vi "ER2007 Take Data Popup Panel.vi"() -> ()   [LabVIEW 2013]
uses:
  Controls/Global ER2007.vi
panel:
  in  "Comment":string
  in  "Delta P :":dbl format="%.2f"
  in  "Mark Options":T1(radio)
  in  "OK":bool
  in  "Pore Volume :":dbl format="%.4f"
  out "Amplitude :":dbl format="%.1f"
  out "Frequency :":dbl format="%#_0f"
  in  "Cancel":bool
  out "Cell Number :":string="<none>"
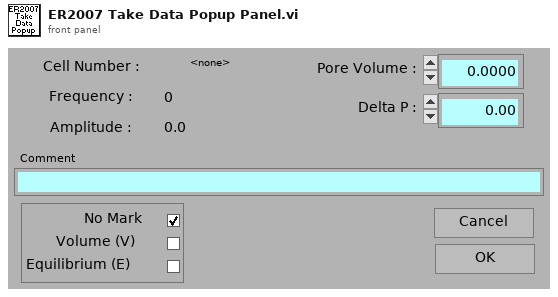
[diagram p1: front panel]
types:
  T1 = enum32{"No Mark", "Volume (V)", "Equilibrium (E)"}
  T2 = cluster{"CurCell":i32, "Cell Data":cluster{"Cell ID":i32, "Cell Status":enum16{"Inactive", "Setup", "Active", "Done"}, "Project":string, "Sample #":string, "Rock Type":string, "Fluid Pair":string, "Rw":dbl, "Rw Temp":dbl, "Length":dbl, "Diameter":dbl, "Porosity":dbl, "Permeability":dbl, "4P":bool, "ElectSpace":dbl, "Frequency":dbl, "Amplitude":dbl, "DAQ Period":u32, "DAQ Units":u16, "Start Time":dbl, "Next Time":dbl, "Datafile":path, "Last Pore Vol":dbl, "Last Pore Xdcr":enum16{"<none>", "Lo Range", "Hi Range"}, "Last Resistor":enum16{"<none>", "Resistor 1", "Resistor 2", "Resistor 3", "Resistor 4", "Resistor 5", "Resistor 6"}, "CurData":dbl[][], "Comment":string}[]}
  T3 = cluster{"Cell ID":i32, "Cell Status":enum16{"Inactive", "Setup", "Active", "Done"}, "Project":string, "Sample #":string, "Rock Type":string, "Fluid Pair":string, "Rw":dbl, "Rw Temp":dbl, "Length":dbl, "Diameter":dbl, "Porosity":dbl, "Permeability":dbl, "4P":bool, "ElectSpace":dbl, "Frequency":dbl, "Amplitude":dbl, "DAQ Period":u32, "DAQ Units":u16, "Start Time":dbl, "Next Time":dbl, "Datafile":path, "Last Pore Vol":dbl, "Last Pore Xdcr":enum16{"<none>", "Lo Range", "Hi Range"}, "Last Resistor":enum16{"<none>", "Resistor 1", "Resistor 2", "Resistor 3", "Resistor 4", "Resistor 5", "Resistor 6"}, "CurData":dbl[][], "Comment":string}[]
  T4 = cluster{"Cell ID":i32, "Cell Status":enum16{"Inactive", "Setup", "Active", "Done"}, "Project":string, "Sample #":string, "Rock Type":string, "Fluid Pair":string, "Rw":dbl, "Rw Temp":dbl, "Length":dbl, "Diameter":dbl, "Porosity":dbl, "Permeability":dbl, "4P":bool, "ElectSpace":dbl, "Frequency":dbl, "Amplitude":dbl, "DAQ Period":u32, "DAQ Units":u16, "Start Time":dbl, "Next Time":dbl, "Datafile":path, "Last Pore Vol":dbl, "Last Pore Xdcr":enum16{"<none>", "Lo Range", "Hi Range"}, "Last Resistor":enum16{"<none>", "Resistor 1", "Resistor 2", "Resistor 3", "Resistor 4", "Resistor 5", "Resistor 6"}, "CurData":dbl[][], "Comment":string}
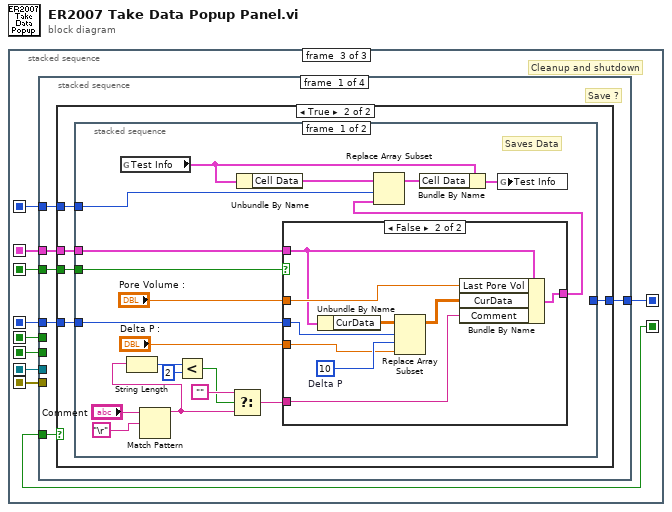
[diagram p0: block diagram]
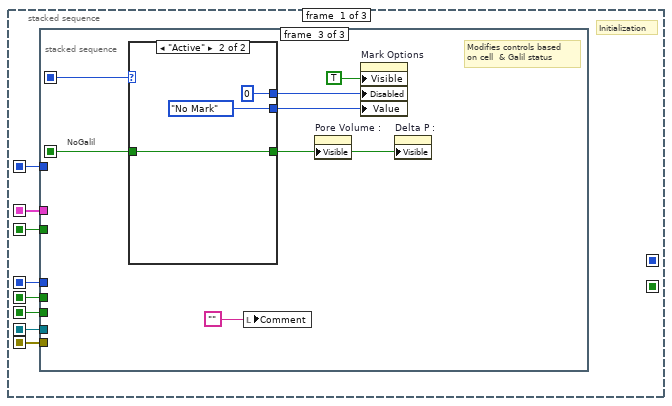
[diagram p2: hidden frame]
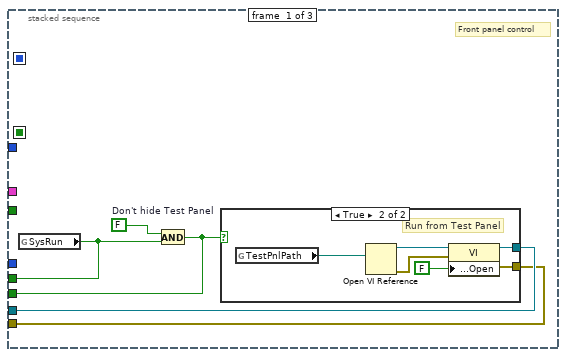
[diagram p3: hidden frame]
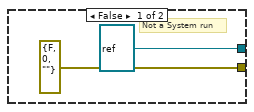
[diagram p4: hidden frame]
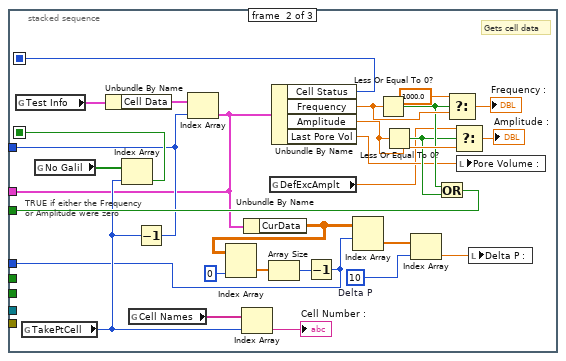
[diagram p5: hidden frame]
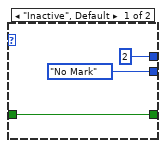
[diagram p6: hidden frame]
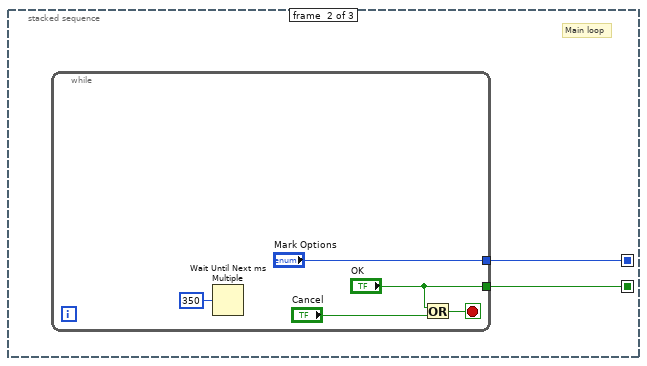
[diagram p7: hidden frame]
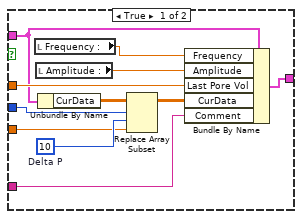
[diagram p9: hidden frame]
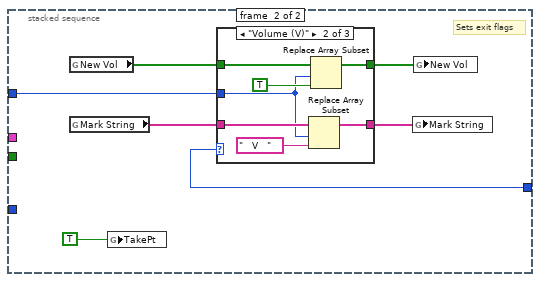
[diagram p10: hidden frame]
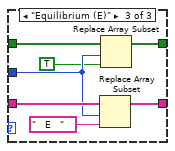
[diagram p12: hidden frame]
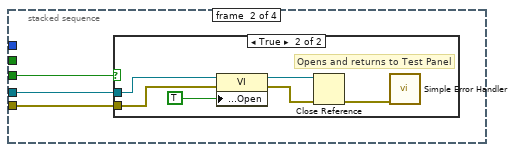
[diagram p13: hidden frame]
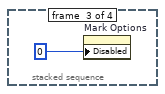
[diagram p15: hidden frame]
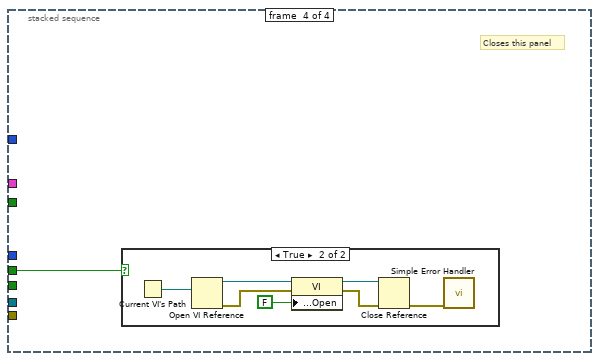
[diagram p16: hidden frame]
diagram:
  n1 = stacked-sequence {
    seq-local: [_ w64 _] -> [_ _ w77]
    seq-local: [w8 _ _] -> [_ _ w79]
    seq-local: [w7 _ _] -> [_ _ w78]
    seq-local: [w6 _ _] -> [_ _ w74]
    seq-local: [w5 _ _] -> [_ _ w75]
    seq-local: [w4 _ _] -> [_ _ w76]
    seq-local: [w3 _ _] -> [_ _ w73]
    seq-local: [w2 _ _] -> [_ _ w72]
    seq-local: [_ w63 _] -> [_ _ w71]
    seq-local: [w1 _ _] -> [_ _ w70]
    frame #0 {
      # "Initialization"
      n2 = stacked-sequence {
        seq-local: [_ w39 _] -> [_ _ w56]
        seq-local: [_ w33 _] -> [_ _ w55]
        tunnel: [_ w30 _] -> w8
        tunnel: [_ w31 _] -> w7
        tunnel: [w11 _ _] -> w6
        tunnel: [w13 _ _] -> w5
        tunnel: [w12 _ _] -> w4
        tunnel: [_ w41 _] -> w3
        tunnel: [w9 _ _] -> w2
        tunnel: [_ w22 _] -> w1
        frame #0 {
          w10 = FALSE  # Don't hide Test Panel
          # "Front panel control"
          n3 = global read "Global ER2007.vi" "SysRun"() -> (w9:bool)
          n4 = And(x=w10, y=w9) -> (x .and. y?=w11:bool)
          n5 = case shown="True" w11 {
            tunnel: [refnum<vi> refnum w18] -> w13
            tunnel: [errorcluster {"status"=FALSE, "code"=0, "source"=""} ("error out") w17] -> w12
            frame False {
              # "Not a System run"
            }
            frame True {
              # "Run from Test Panel"
              n6 = global read "Global ER2007.vi" "TestPnlPath"() -> (w16:path)
              n7 = Open VI Reference(vi path=w16) -> (vi reference=w21:refnum<vi>, error out=w20:errorcluster)  [unwired: 5 in]
              n8 = property class="VI"(reference=w21, error in=w20, "Front Panel Window:Open"=FALSE) -> (reference out=w18:refnum<vi>, error out=w17:errorcluster)
            }
          }
        }
        frame #1 {
          w24 = 10  # Delta P
          # "Gets cell data"
          # "TRUE if either the Frequency\nor Amplitude were zero"
          n9 = global read "Global ER2007.vi" "Test Info"() -> (w38:T2)
          n10 = global read "Global ER2007.vi" "TakePtCell"() -> (w32:i32)
          n11 = global read "Global ER2007.vi" "No Galil"() -> (w34:bool[])
          n12 = Unbundle By Name(w38) -> ("Cell Data"=w49:T3)
          n13 = Index Array(array=w34, index=w32) -> (element=w33:bool)
          n14 = global read "Global ER2007.vi" "Cell Names"() -> (w36:string[])
          n15 = Decrement(x=w32) -> (x-1=w31:i32)
          n16 = Index Array(array=w49, index=w31) -> (element=w30:T4)
          n17 = Index Array(array=w36, index=w32) -> (element=→"Cell Number :":string)
          n18 = Unbundle By Name(w30) -> ("CurData"=w26:dbl[][])
          n19 = Index Array(array=w26, index (col)=0 ("disabled index (col)")) -> (element=w28:dbl[])  [unwired: 1 in]
          n20 = Array Size(array=w28) -> (size(s)=w27:i32)
          n21 = global read "Global ER2007.vi" "DefExcAmplt"() -> (w37:dbl)
          n22 = Unbundle By Name(w30) -> ("Cell Status"=w39:enum16{"Inactive", "Setup", "Active", "Done"}, "Frequency"=w46:dbl, "Amplitude"=w48:dbl, "Last Pore Vol"=w40:dbl)
          n23 = Decrement(x=w27) -> (x-1=w22:i32)
          n24 = Index Array(array=w26, index (row)=w22) -> (element=w25:dbl[])  [unwired: 1 in]
          n25 = Less Or Equal To 0?(x=w46) -> (x <= 0?=w43:bool)
          n26 = Less Or Equal To 0?(x=w48) -> (x <= 0?=w42:bool)
          n27 = Index Array(array=w25, index=w24) -> (element=w23:dbl)
          n28 = Or(x=w43, y=w42) -> (x .or. y?=w41:bool)
          n29 = Select(t=1000.0, s=w43, f=w46) -> (s? t:f=→"Frequency :":dbl)
          n30 = Select(t=w37, s=w42, f=w48) -> (s? t:f=→"Amplitude :":dbl)
          n31 = local write "Pore Volume :"(w40) -> ()
          n32 = local write "Delta P :"(w23) -> ()
        }
        frame #2 {
          # "NoGalil"
          # "Modifies controls based\non cell  & Galil status"
          n33 = case shown="\"Active\"" w56 {
            tunnel: [u8 2 ("Disabled") u8 0 ("Disabled")] -> w53
            tunnel: w55 -> [w58 w61]
            tunnel: [w58 w61] -> w54
            tunnel: [T1."No Mark" ("Mark Options") T1."No Mark" ("Mark Options")] -> w52
            frame "Inactive", Default {
            }
            frame "Active" {
            }
          }
          n34 = local write "Comment"("") -> ()
          n35 = property on="Pore Volume :" class="DigNum (strict)"("Visible"=w54) -> ()  [unwired: 2 in, 2 out]
          n36 = property on="Mark Options" class="RadioBtnsControl (strict)"("Visible"=TRUE, "Disabled"=w53, "Value"=w52) -> ()  [unwired: 2 in, 2 out]
          n37 = property on="Delta P :" class="DigNum (strict)"("Visible"=w54) -> ()  [unwired: 2 in, 2 out]
        }
      }
    }
    frame #1 {
      # "Main loop"
      n38 = while {
        tunnel: ["OK"] -> w64
        tunnel: ["Mark Options"] -> w63
        stop <- w67 stop-if-true
        n39 = Wait Until Next ms Multiple(millisecond multiple=u32 350) -> ()  [unwired: 1 out]
        n40 = Or(x="OK", y="Cancel") -> (x .or. y?=w67:bool)
      }
    }
    frame #2 {
      # "Cleanup and shutdown"
      n41 = stacked-sequence {
        tunnel: w77 -> [w85 _ _ _]
        tunnel: w79 -> [w84 _ _ _]
        tunnel: w78 -> [w83 _ _ _]
        tunnel: w76 -> [_ w155 _ _]
        tunnel: w75 -> [_ w154 _ _]
        tunnel: w74 -> [_ w153 _ _]
        tunnel: w73 -> [w82 _ _ _]
        tunnel: w72 -> [_ _ _ w163]
        tunnel: w71 -> [w81 _ _ _]
        tunnel: w70 -> [w80 _ _ _]
        frame #0 {
          # "Save ?"
          n42 = case shown="True" w85 {
            tunnel: w84 -> [_ w90]
            tunnel: w83 -> [_ w89]
            tunnel: w82 -> [_ w88]
            tunnel: w81 -> [_ w87]
            tunnel: w80 -> [_ w86]
            frame False {
            }
            frame True {
              n43 = stacked-sequence {
                tunnel: w90 -> [w101 _]
                tunnel: w89 -> [w109 w130]
                tunnel: w88 -> [w107 _]
                tunnel: w87 -> [_ w135]
                tunnel: w86 -> [w100 _]
                frame #0 {
                  # "Saves Data"
                  n44 = global read "Global ER2007.vi" "Test Info"() -> (w103:T2)
                  n45 = Match Pattern(string="Comment", regular expression="\r") -> (before substring=w97:string)  [unwired: 1 in, 3 out]
                  n46 = String Length(string=w97) -> (length=w93:i32)
                  n47 = Less?(x=w93, y=2) -> (x < y?=w96:bool)
                  n48 = Select(t="", s=w96, f=w97) -> (s? t:f=w91:string)
                  n49 = Unbundle By Name(w103) -> ("Cell Data"=w105:T3)
                  n50 = case shown="False" w107 {
                    tunnel: w101 -> [w116 w125]
                    tunnel: [w120 w129] -> w102
                    tunnel: "Pore Volume :" -> [w119 w128]
                    tunnel: w100 -> [w113 w124]
                    tunnel: "Delta P :" -> [w112 w123]
                    tunnel: w91 -> [w110 w121]
                    frame True {
                      w114 = 10  # Delta P
                      n51 = local read "Frequency :"() -> (w118:dbl)
                      n52 = local read "Amplitude :"() -> (w117:dbl)
                      n53 = Unbundle By Name(w116) -> ("CurData"=w115:dbl[][])
                      n54 = Replace Array Subset(array=w115, new element=w112, index (row)=w113, index (col)=w114) -> (w111:dbl[][])
                      n55 = Bundle By Name(cluster=w116, "Frequency"=w118, "Amplitude"=w117, "Last Pore Vol"=w119, "CurData"=w111, "Comment"=w110) -> (w120:T4)
                    }
                    frame False {
                      w126 = 10  # Delta P
                      n56 = Unbundle By Name(w125) -> ("CurData"=w127:dbl[][])
                      n57 = Replace Array Subset(array=w127, new element=w123, index (row)=w124, index (col)=w126) -> (w122:dbl[][])
                      n58 = Bundle By Name(cluster=w125, "Last Pore Vol"=w128, "CurData"=w122, "Comment"=w121) -> (w129:T4)
                    }
                  }
                  n59 = Replace Array Subset(array=w105, new element=w102, index=w109) -> (w108:T3)
                  n60 = Bundle By Name(cluster=w103, "Cell Data"=w108) -> (w104:T2)
                  n61 = global write "Global ER2007.vi" "Test Info"(w104) -> ()
                }
                frame #1 {
                  # "Sets exit flags"
                  n62 = global read "Global ER2007.vi" "New Vol"() -> (w132:bool[])
                  n63 = global read "Global ER2007.vi" "Mark String"() -> (w131:string[])
                  n64 = global write "Global ER2007.vi" "TakePt"(TRUE ("New Setup")) -> ()
                  n65 = case shown="\"Volume (V)\"" w135 {
                    tunnel: [w138 w143 w149] -> w134
                    tunnel: [w137 w141 w151] -> w133
                    tunnel: w132 -> [w138 w145 w150]
                    tunnel: w131 -> [w137 w142 w152]
                    tunnel: w130 -> [_ w140 w148]
                    frame "No Mark", Default {
                    }
                    frame "Volume (V)" {
                      n66 = Replace Array Subset(array=w142, new element="   V   ", index=w140) -> (w141:string[])
                      n67 = Replace Array Subset(array=w145, new element=TRUE, index=w140) -> (w143:bool[])
                    }
                    frame "Equilibrium (E)" {
                      n68 = Replace Array Subset(array=w152, new element="   E   ", index=w148) -> (w151:string[])
                      n69 = Replace Array Subset(array=w150, new element=TRUE, index=w148) -> (w149:bool[])
                    }
                  }
                  n70 = global write "Global ER2007.vi" "Mark String"(w133) -> ()
                  n71 = global write "Global ER2007.vi" "New Vol"(w134) -> ()
                }
              }
            }
          }
        }
        frame #1 {
          n72 = case shown="True" w153 {
            tunnel: w154 -> [_ w156]
            tunnel: w155 -> [_ w157]
            frame False {
            }
            frame True {
              # "Opens and returns to Test Panel"
              n73 = property class="VI"(reference=w156, error in=w157, "Front Panel Window:Open"=TRUE) -> (reference out=w160:refnum<vi>, error out=w159:errorcluster)
              n74 = Close Reference(reference=w160, error in (no error)=w159) -> (error out=w158:errorcluster)
              n75 = call <vilib>:"Simple Error Handler.vi"("error in (no error)"=w158) -> ()  [unwired: 4 in, 5 out]
            }
          }
        }
        frame #2 {
          n76 = property on="Mark Options" class="RadioBtnsControl (strict)"("Disabled"=u8 0) -> ()  [unwired: 2 in, 2 out]
        }
        frame #3 {
          # "Closes this panel"
          n77 = case shown="True" w163 {
            frame False {
            }
            frame True {
              n78 = Current VI's Path() -> (path=w170:path)
              n79 = Open VI Reference(vi path=w170) -> (vi reference=w169:refnum<vi>, error out=w168:errorcluster)  [unwired: 5 in]
              n80 = property class="VI"(reference=w169, error in=w168, "Front Panel Window:Open"=FALSE) -> (reference out=w166:refnum<vi>, error out=w165:errorcluster)
              n81 = Close Reference(reference=w166, error in (no error)=w165) -> (error out=w164:errorcluster)
              n82 = call <vilib>:"Simple Error Handler.vi"("error in (no error)"=w164) -> ()  [unwired: 4 in, 5 out]
            }
          }
        }
      }
    }
  }
